vi "UIQ_FGV.vi"(7 "Enum":enum16{"Initial", "Write", "Read"}(ring)=enum."Read", 10 "DataIn":variant, 11 "Index":i32) -> (2 "DataOut":variant)   [LabVIEW 2019]
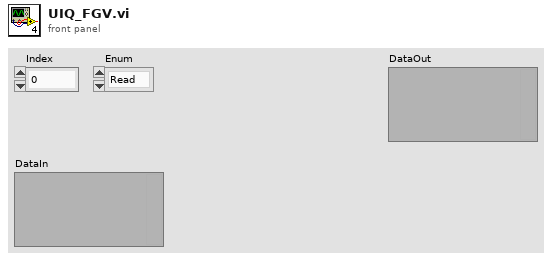
[diagram p1: front panel]
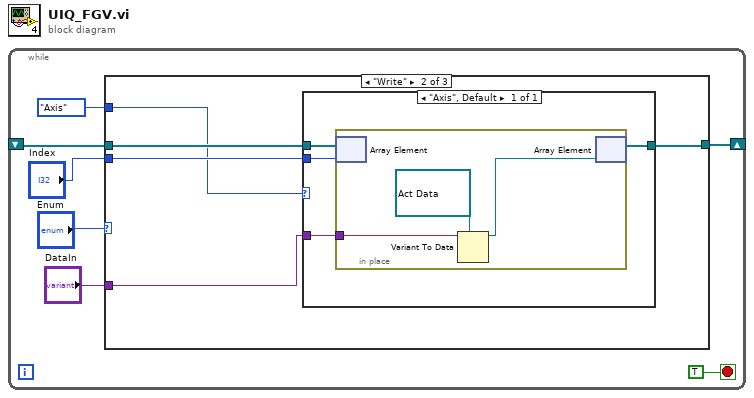
[diagram p0: block diagram]
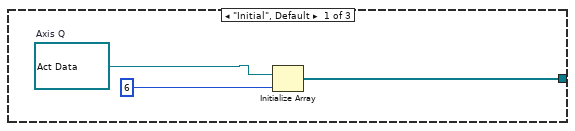
[diagram p2: hidden frame]
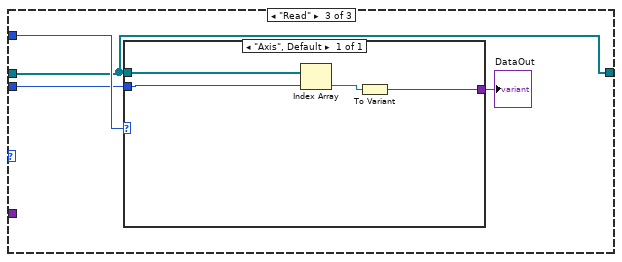
[diagram p3: hidden frame]
diagram:
  n1 = while {
    shift-right: [w6] -> _
    shift-left: _ -> [w5]
    stop <- TRUE stop-if-true
    n2 = case shown="\"Write\"" "Enum" {
      tunnel: [w8 w14 w25] -> w6
      tunnel: w5 -> [_ w13 w25]
      tunnel: "Index" -> [_ w15 w24]
      tunnel: "DataIn" -> [_ w12 _]
      tunnel: enum16{"Axis"}."Axis" -> [_ w11 w26]
      frame "Initial", Default {
        w10 = refnum<queue> refnum  # Axis Q
        n3 = Initialize Array(w10, 6 ("dimension size")) -> (w8:refnum<queue>[])
      }
      frame "Write" {
        n4 = case shown="\"Axis\", Default" w11 {
          tunnel: w15 -> [w19]
          tunnel: [w18] -> w14
          tunnel: w13 -> [w17]
          tunnel: w12 -> [w16]
          frame "Axis", Default {
            n5 = in-place {
              in-place-border: w16 -> [w21]
              n6 = in-place-array #1(w17, w19) -> ()  [unwired: 1 out]
              n7 = Variant To Data(type=refnum<queue> refnum ("Axis Q"), Variant=w21) -> (data=w20:refnum<queue>)  [unwired: 1 in, 1 out]
              n8 = in-place-array #1(w20) -> (w18:refnum<queue>[])  [unwired: 1 out]
            }
          }
        }
      }
      frame "Read" {
        n9 = case shown="\"Axis\", Default" w26 {
          tunnel: w25 -> [w30]
          tunnel: w24 -> [w29]
          tunnel: [w27] -> w23
          frame "Axis", Default {
            n10 = Index Array(array=w30, index=w29) -> (element=w28:refnum<queue>)
            n11 = To Variant(anything=w28) -> (Variant=w27:variant)
          }
        }
        "DataOut" <- w23
      }
    }
  }
